vi "_ROSMasterConsole.vi"() -> ()   [LabVIEW 2012]
uses:
  <vilib>/Utility/miscctls.llb/LVRectTypeDef.ctl
  <userlib>/ROSforLV/ROS/Code/_ROSDefinition.vi
  <vilib>/Utility/cursorutil.llb/Set Cursor (Icon Pict).vi
panel:
  out "Servers Closed":bool[](array[boolean])
  in  "Stop":bool
  out "Error Log":string
  out "ROS Master":string="192.168.1.110:11311"
  out "selection":i32=-1
  out "2D Picture":picture
  out "Boundaries":cluster{i32, i32}[](array[cluster])=[{10, 22}, {30, 42}, {50, 62}]
  in  "expand?":bool
  out "Status":string
  out "Master?":bool
  out "Running?":bool
  out "current task":string
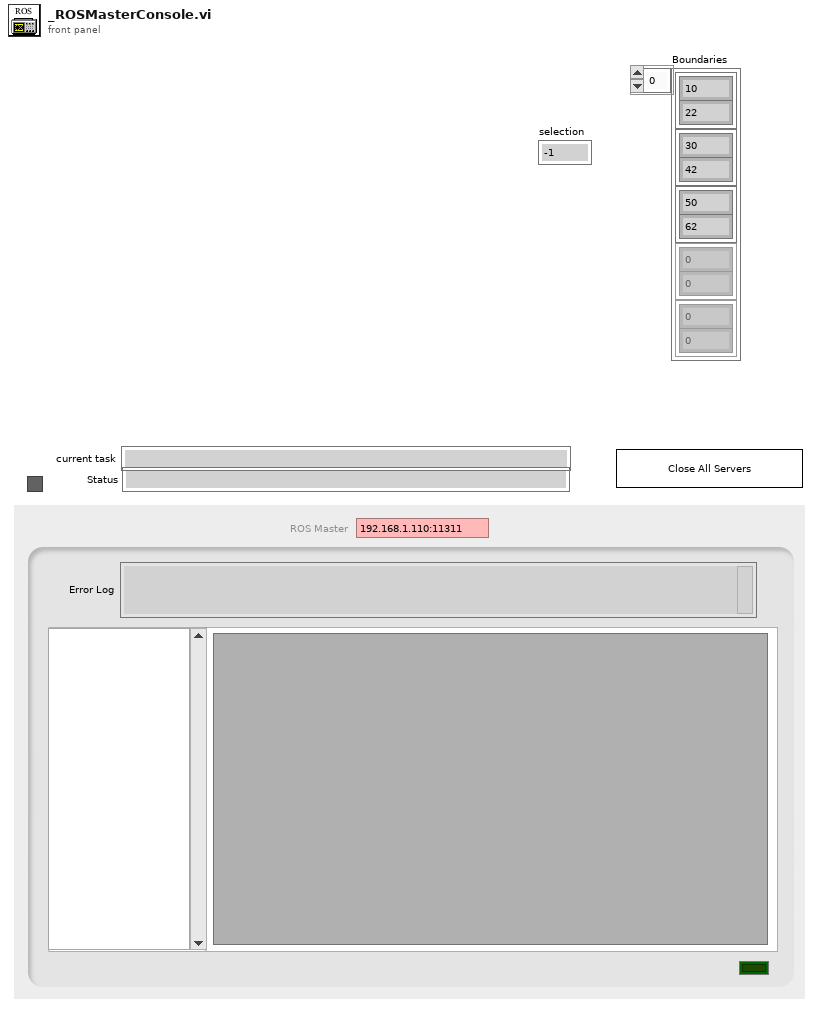
[diagram p1: front panel]
types:
  T1 = enum16{"Add Server", "Clear Server", "Clear All", "Get Info"}
  T2 = enum16{"Get Nodes", "Start Nodes", "Reset Nodes"}
  T3 = typedef "LVRectTypeDef.ctl" = cluster{"Left":i16, "Top":i16, "Right":i16, "Bottom":i16}
  T4 = typedef "_ROSControl.ctl" = cluster{"topic port":u16, "Node":string, "topic":string, "type":string, "node port":u32, "error ":errorcluster, "Direction":T5, "APIs":string[], "Update (ms)":u16, "write queue":u16}
  T5 = typedef "_ROSDirection.ctl" = enum16{"Node", "Publisher", "Subscriber", "Service Client"}
  T6 = typedef "ServoInfo.ctl" = cluster{"vi name":string, "VI Refnum":refnum<vi>, "queue":refnum<queue>, "ROS":T4, "notifier":refnum<notifier>}
  T7 = typedef "LVMouseTypeDef.ctl" = cluster{"Mouse Position":cluster{"X":i32, "Y":i32}, "Mouse Modifiers":cluster{"Button Down":bool, "Shift Mod":bool, "Menu Mod":bool, "Option Mod":bool}}
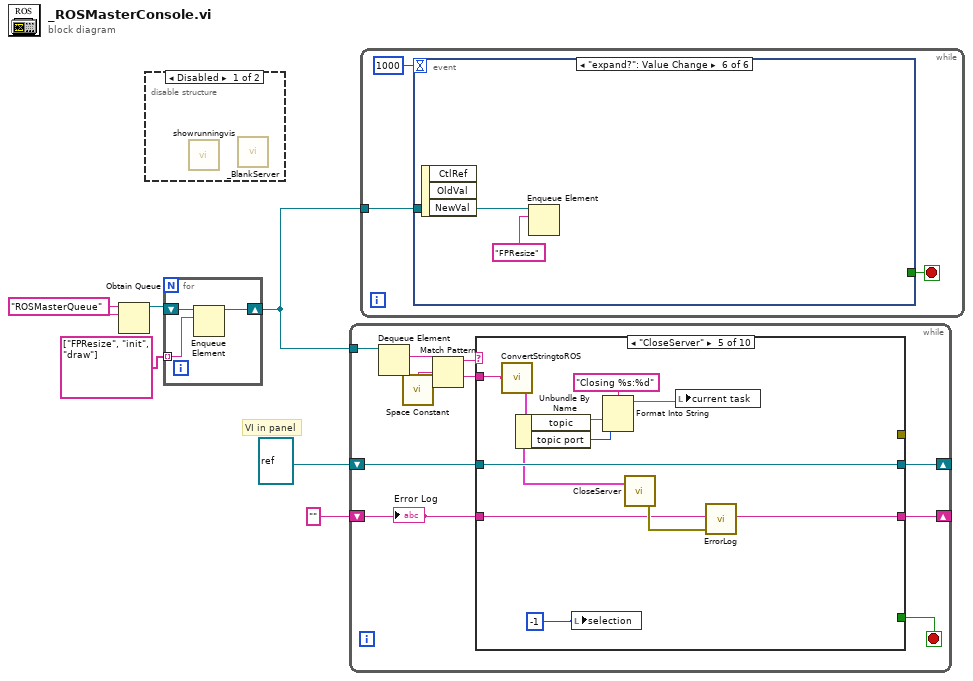
[diagram p0: block diagram]
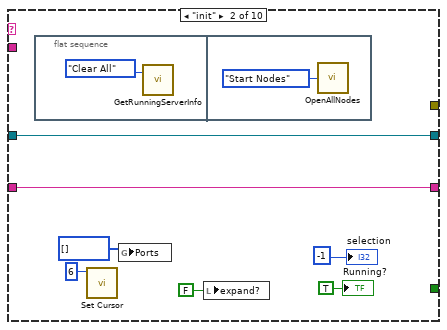
[diagram p4: hidden frame]
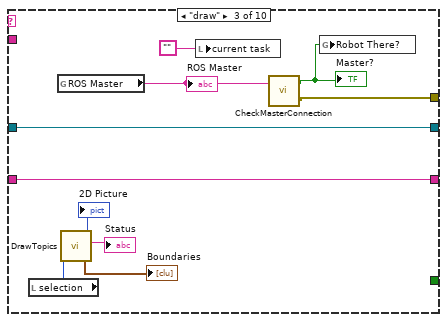
[diagram p5: hidden frame]
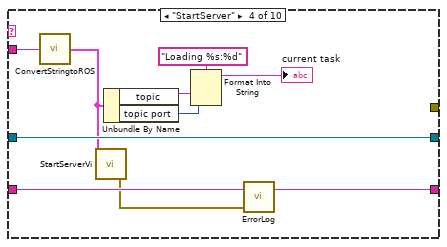
[diagram p6: hidden frame]
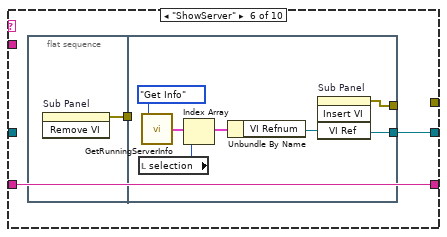
[diagram p7: hidden frame]
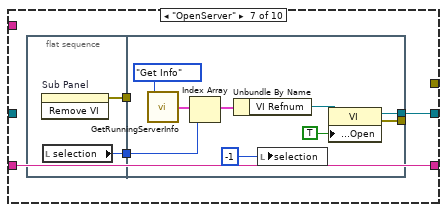
[diagram p8: hidden frame]
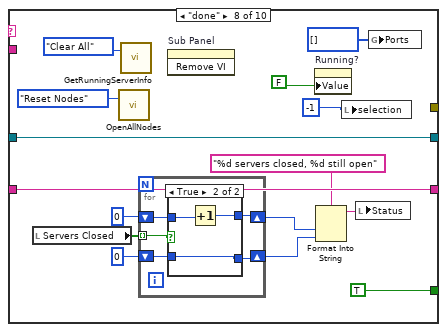
[diagram p9: hidden frame]
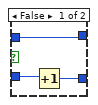
[diagram p10: hidden frame]
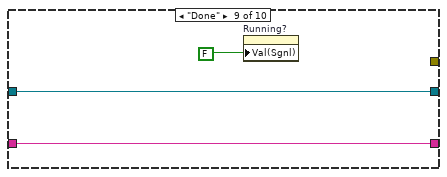
[diagram p11: hidden frame]
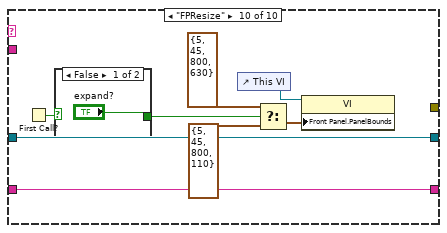
[diagram p12: hidden frame]
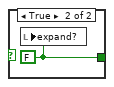
[diagram p13: hidden frame]
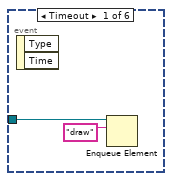
[diagram p14: hidden frame]
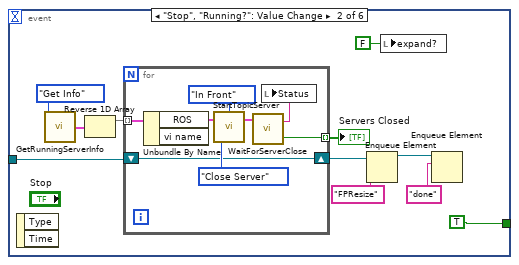
[diagram p15: hidden frame]
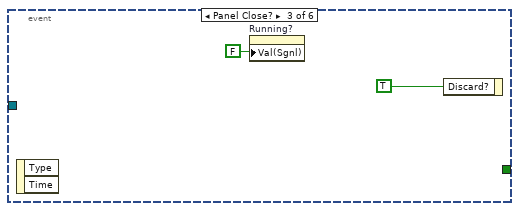
[diagram p16: hidden frame]
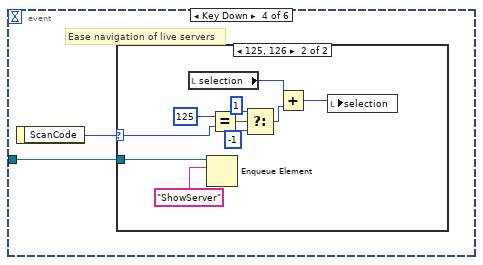
[diagram p17: hidden frame]
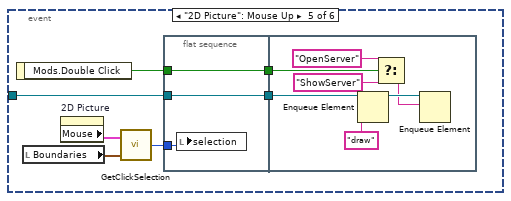
[diagram p19: hidden frame]
diagram:
  w6 = "ROSMasterQueue" ("name (unnamed)")
  # "VI in panel"
  n1 = Obtain Queue(name (unnamed)=w6, element data type=w6) -> (queue out=w3:refnum<queue>)  [unwired: 3 in, 2 out]
  n2 = disable-structure shown="Disabled" {
    frame Disabled {
      n3 = call <userlib>:"showrunningvis.vi"() -> ()  [unwired: 1 in]
      n4 = call <userlib>:"_BlankServer.vi"() -> ()  [unwired: 4 in]
    }
    frame Enabled {
    }
  }
  n5 = for {
    shift-right: [w9] -> w5
    shift-left: w3 -> [w8]
    tunnel: string[] ["FPResize", "init", "draw"] -> [w7] mode=indexing
    n6 = Enqueue Element(queue=w8, element=w7) -> (queue out=w9:refnum<queue>)  [unwired: 2 in, 2 out]
  }
  n7 = while {
    tunnel: w5 -> [w19]
    shift-right: [w12] -> _
    shift-left: refnum<vi> refnum ("VI Ref") -> [w13]
    shift-right: [w11] -> _
    shift-left: "" ("String out") -> [w10]
    stop <- w18 stop-if-true
    n8 = Dequeue Element(queue=w19) -> (element=w16:string)  [unwired: 2 in, 3 out]
    n9 = call <vilib>:"Space Constant.vi"() -> ("String"=w15:string)
    n10 = Match Pattern(string=w16, regular expression=w15) -> (before substring=w17:string, after substring=w14:string)  [unwired: 1 in, 2 out]
    n11 = case shown="\"CloseServer\"" w17 {
      tunnel: [_ _ _ _ _ _ _ TRUE _ _] -> w18
      tunnel: w14 -> [_ _ _ w47 w53 _ _ _ _ _]
      tunnel: w13 -> [w21 w28 w40 w50 w61 _ _ w100 w115 w123]
      tunnel: [w21 w28 w40 w50 w61 w63 w73 w100 w115 w123] -> w12
      tunnel: [_ _ w34 _ _ _ _ _ _ _] -> _
      tunnel: [w20 w22 w36 w42 w57 w62 w72 w95 w113 w116] -> w11
      tunnel: w10 -> [w20 w22 w36 w43 w58 w62 w72 w95 w113 w116]
      frame Default {
      }
      frame "init" {
        n12 = flat-sequence {
          frame #0 {
            n13 = call <userlib>:"GetRunningServerInfo.vi"("Task"=T1."Clear All") -> ()  [unwired: 1 in, 3 out]
          }
          frame #1 {
            n14 = call <userlib>:"OpenAllNodes.vi"("Task"=T2."Start Nodes") -> ()  [unwired: 1 in, 1 out]
          }
        }
        n15 = call-poly <vilib>:"Set Cursor.vi"("icon"=u16 6) -> ()  [unwired: 9 in, 2 out]
        n16 = global write "_ROSDefinition.vi" "Ports"(u16[] [] ("Ports")) -> ()
        n17 = local write "expand?"(FALSE ("expand?")) -> ()
        "Running?" <- TRUE ("Running?")
        "selection" <- -1 ("selection")
      }
      frame "draw" {
        n18 = local read "selection"() -> (w39:i32)
        n19 = global read "_ROSDefinition.vi" "ROS Master"() -> (w33:string)
        "ROS Master" <- w33
        n20 = call <userlib>:"DrawTopics.vi"("Selection"=w39) -> ("new picture"=→"2D Picture":picture, "Status"=→"Status":string, "Boundaries"=→"Boundaries":cluster{i32, i32}[])  [unwired: 2 in, 1 out]
        n21 = local write "current task"("") -> ()
        n22 = call <userlib>:"CheckMasterConnection.vi"("Master IP"=w33) -> ("error out"=w34:errorcluster, "Master There?"=w31:bool)  [unwired: 1 in]
        "Master?" <- w31
        n23 = global write "_ROSDefinition.vi" "Robot There?"(w31) -> ()
      }
      frame "StartServer" {
        n24 = call <userlib>:"ConvertStringtoROS.vi"("string in"=w47) -> ("ROS"=w44:T4)
        n25 = call <userlib>:"StartServerVi.vi"("ROS in"=w44) -> ("error out"=w41:errorcluster)  [unwired: 2 out]
        n26 = Unbundle By Name(w44) -> ("topic"=w46:string, "topic port"=w45:u16)
        n27 = Format Into String(format string="Loading %s:%d", w46, w45) -> (resulting string=→"current task":string)  [unwired: 2 in, 1 out]
        n28 = call <userlib>:"ErrorLog.vi"("error in"=w41, "String in"=w43) -> ("String out"=w42:string)  [unwired: 1 in, 1 out]
      }
      frame "CloseServer" {
        n29 = call <userlib>:"ConvertStringtoROS.vi"("string in"=w53) -> ("ROS"=w51:T4)
        n30 = Unbundle By Name(w51) -> ("topic"=w55:string, "topic port"=w54:u16)
        n31 = local write "selection"(-1 ("Value (Signaling)")) -> ()
        n32 = Format Into String(format string="Closing %s:%d", w55, w54) -> (resulting string=w52:string)  [unwired: 2 in, 1 out]
        n33 = call <userlib>:"CloseServer.vi"("ROS"=w51) -> ("error out"=w59:errorcluster)  [unwired: 2 in]
        n34 = local write "current task"(w52) -> ()
        n35 = call <userlib>:"ErrorLog.vi"("error in"=w59, "String in"=w58) -> ("String out"=w57:string)  [unwired: 1 in, 1 out]
      }
      frame "ShowServer" {
        n36 = flat-sequence {
          tunnel: [w65] -> w64
          tunnel: w64 -> [_]
          tunnel: [w71] -> _
          tunnel: [w66] -> w63
          frame #0 {
            n37 = invoke on="Sub Panel" class="SubPanel" method="Remove VI"() -> (error out=w65:errorcluster)  [unwired: 3 in, 2 out]
          }
          frame #1 {
            n38 = local read "selection"() -> (w70:i32)
            n39 = call <userlib>:"GetRunningServerInfo.vi"("Task"=T1."Get Info") -> ("servers"=w68:T6[])  [unwired: 1 in, 2 out]
            n40 = Index Array(array=w68, index=w70) -> (element=w67:T6)
            n41 = Unbundle By Name(w67) -> ("VI Refnum"=w66:refnum<vi>)
            n42 = invoke on="Sub Panel" class="SubPanel" method="Insert VI"("VI Ref"=w66) -> (error out=w71:errorcluster)  [unwired: 3 in, 3 out]
          }
        }
      }
      frame "OpenServer" {
        n43 = flat-sequence {
          tunnel: [w77] -> w75
          tunnel: [w76] -> w74
          tunnel: w75 -> [_]
          tunnel: w74 -> [w79]
          tunnel: [w84] -> w73
          tunnel: [w83] -> _
          frame #0 {
            n44 = invoke on="Sub Panel" class="SubPanel" method="Remove VI"() -> (error out=w77:errorcluster)  [unwired: 3 in, 2 out]
            n45 = local read "selection"() -> (w76:i32)
          }
          frame #1 {
            n46 = call <userlib>:"GetRunningServerInfo.vi"("Task"=T1."Get Info") -> ("servers"=w81:T6[])  [unwired: 1 in, 2 out]
            n47 = Index Array(array=w81, index=w79) -> (element=w80:T6)
            n48 = Unbundle By Name(w80) -> ("VI Refnum"=w78:refnum<vi>)
            n49 = local write "selection"(-1 ("Live Servers")) -> ()
            n50 = property class="VI"(reference=w78, "Front Panel.Open"=TRUE ("Front Panel Window:Open")) -> (reference out=w84:refnum<vi>, error out=w83:errorcluster)  [unwired: 1 in]
          }
        }
      }
      frame "done" {
        n51 = local read "Servers Closed"() -> (w94:bool[])
        n52 = call <userlib>:"OpenAllNodes.vi"("Task"=T2."Reset Nodes") -> ()  [unwired: 1 in, 1 out]
        n53 = call <userlib>:"GetRunningServerInfo.vi"("Task"=T1."Clear All") -> ()  [unwired: 1 in, 3 out]
        n54 = for {
          shift-right: [w104] -> w90
          shift-left: 0 -> [w105]
          shift-right: [w102] -> w89
          shift-left: 0 -> [w103]
          tunnel: w94 -> [w106] mode=indexing
          n55 = case shown="True" w106 {
            tunnel: w105 -> [w107 w112]
            tunnel: [w107 w111] -> w104
            tunnel: w103 -> [w109 w110]
            tunnel: [w108 w110] -> w102
            frame False {
              n56 = Increment(x=w109) -> (x+1=w108:i32)
            }
            frame True {
              n57 = Increment(x=w112) -> (x+1=w111:i32)
            }
          }
        }
        n58 = invoke on="Sub Panel" class="SubPanel" method="Remove VI"() -> ()  [unwired: 3 in, 3 out]
        n59 = property on="Running?" class="Bool (strict)"("Value"=FALSE) -> ()  [unwired: 2 in, 2 out]
        n60 = Format Into String(format string="%d servers closed, %d still open", w90, w89) -> (resulting string=w88:string)  [unwired: 2 in, 1 out]
        n61 = local write "selection"(-1 ("Live Servers")) -> ()
        n62 = local write "Status"(w88) -> ()
        n63 = global write "_ROSDefinition.vi" "Ports"(u16[] [] ("Ports")) -> ()
      }
      frame "Done" {
        n64 = property on="Running?" class="Bool (strict)"("Val(Sgnl)"=FALSE) -> ()  [unwired: 2 in, 2 out]
      }
      frame "FPResize" {
        n65 = First Call?() -> (First Call?: T/F=w118:bool)
        n66 = case shown="False" w118 {
          tunnel: ["expand?" w125] -> w117
          frame False {
          }
          frame True {
            w125 = FALSE ("expand?")
            n67 = local write "expand?"(w125) -> ()
          }
        }
        n68 = control-ref of="This VI"() -> (w122:refnum<vi>)
        n69 = Select(t=T3 {"Left"=5, "Top"=45, "Right"=800, "Bottom"=630} ("Front Panel Window:Panel Bounds"), s=w117, f=T3 {"Left"=5, "Top"=45, "Right"=800, "Bottom"=110} ("Front Panel Window:Panel Bounds")) -> (s? t:f=w120:T3)
        n70 = property class="VI"(reference=w122, "Front Panel.PanelBounds"=w120) -> ()  [unwired: 1 in, 2 out]
      }
    }
    "Error Log" <- w10
  }
  n71 = while {
    tunnel: w5 -> [w128]
    stop <- w127 stop-if-true
    n72 = event shown="[5] \"expand?\": Value Change" {
      selector: _ -> [_ _ _ _ _ _]
      dyn-events: _ -> [_ _ _ _ _ _]
      timeout: 1000 -> [_ _ _ _ _ _]
      tunnel: w128 -> [w130 w140 _ w153 w170 w181]
      tunnel: [_ TRUE ("Stop") _ _ _ _] -> w127
      event Timeout {
        n73 = event-data() -> ()  [unwired: 1 in, 2 out]
        n74 = Enqueue Element(queue=w130, element="draw") -> ()  [unwired: 2 in, 3 out]
      }
      event "Stop", "Running?": Value Change {
        n75 = event-data() -> ()  [unwired: 1 in, 2 out]
        n76 = call <userlib>:"GetRunningServerInfo.vi"("Task"=T1."Get Info") -> ("servers"=w132:T6[])  [unwired: 1 in, 2 out]
        n77 = Reverse 1D Array(array=w132) -> (reversed array=w133:T6[])
        n78 = for {
          shift-right: [w145] -> w137
          shift-left: w140 -> [w145]
          tunnel: w133 -> [w149] mode=indexing
          tunnel: [w142] -> w131 mode=indexing
          n79 = Unbundle By Name(w149) -> ("ROS"=w146:T4)  [unwired: 1 out]
          n80 = call <userlib>:"StartTopicServer.vi"("Server Direction"=enum16{"Start Server", "Close Server"}."Close Server", "ROS in"=w146, "Priority"=enum16{"In Front", "In Back"}."In Front") -> ("ROS out"=w144:T4)  [unwired: 1 in]
          n81 = call <userlib>:"WaitForServerClose.vi"("ROS in"=w144) -> ("Closed"=w142:bool, "resulting string"=w143:string)  [unwired: 1 in]
          n82 = local write "Status"(w143) -> ()
        }
        "Servers Closed" <- w131
        n83 = Enqueue Element(queue=w137, element="FPResize") -> (queue out=w136:refnum<queue>)  [unwired: 2 in, 2 out]
        n84 = local write "expand?"(FALSE ("expand?")) -> ()
        n85 = Enqueue Element(queue=w136, element="done") -> ()  [unwired: 2 in, 3 out]
      }
      event Panel Close? {
        n86 = event-data() -> ()  [unwired: 1 in, 2 out]
        n87 = property on="Running?" class="Bool (strict)"("Val(Sgnl)"=FALSE ("Value (Signaling)")) -> ()  [unwired: 2 in, 2 out]
        n88 = event-data("Discard?"=TRUE ("Stop")) -> ()  [unwired: 1 in, 1 out]
      }
      event Key Down {
        # "Ease navigation of live servers"
        n89 = event-data() -> ("ScanCode"=w152:i16)  [unwired: 1 in]
        n90 = case shown="125, 126" w152 {
          selector: w152 -> [_ w161]
          tunnel: w153 -> [_ w163]
          frame Default {
          }
          frame 125, 126 {
            n91 = local read "selection"() -> (w154:i32)
            n92 = Enqueue Element(queue=w163, element="ShowServer") -> ()  [unwired: 2 in, 3 out]
            n93 = Equal?(x=i16 125, y=w161) -> (x = y?=w159:bool)
            n94 = Select(t=i16 1 ("x"), s=w159, f=i16 -1 ("x")) -> (s? t:f=w158:i16)
            n95 = Add(x=w154, y=w158) -> (x+y=w155:i32)
            n96 = local write "selection"(w155) -> ()
          }
        }
      }
      event "2D Picture": Mouse Up {
        n97 = event-data() -> ("Mods.Double Click"=w167:bool)  [unwired: 1 in]
        n98 = local read "Boundaries"() -> (w168:cluster{i32, i32}[])
        n99 = property on="2D Picture" class="Pict"() -> ("Mouse"=w169:T7)  [unwired: 2 in, 2 out]
        n100 = call <userlib>:"GetClickSelection.vi"("Boundaries"=w168, "Mouse"=w169) -> ("selection"=w164:i32)
        n101 = flat-sequence {
          tunnel: w167 -> [w172]
          tunnel: w170 -> [w173]
          tunnel: [w173] -> w166
          tunnel: [w172] -> w165
          tunnel: w164 -> [w171]
          tunnel: w166 -> [w179]
          tunnel: w165 -> [w178]
          frame #0 {
            n102 = local write "selection"(w171) -> ()
          }
          frame #1 {
            n103 = Enqueue Element(queue=w179, element="draw" ("name (unnamed)")) -> (queue out=w175:refnum<queue>)  [unwired: 2 in, 2 out]
            n104 = Select(t="OpenServer" ("element"), s=w178, f="ShowServer" ("element")) -> (s? t:f=w174:string)
            n105 = Enqueue Element(queue=w175, element=w174) -> ()  [unwired: 2 in, 3 out]
          }
        }
      }
      event "expand?": Value Change {
        n106 = event-data() -> ()  [unwired: 1 in, 3 out]
        n107 = Enqueue Element(queue=w181, element="FPResize") -> ()  [unwired: 2 in, 3 out]
      }
    }
  }
